vi "PicoScope2000aNearestSampleInterval.vi"(5 "Enabled array":i16[](array[numeric])=[0, 0, 0, 0, 0, 0, 0, 0, 0, 0], 6 "Acquisition Settings":T1 {"postTriggerSamples" format="%_6p"; "preTriggerSamples" format="%_6p"}, 8 "error in (no error)":errorcluster, 9 "roundFaster":bool, 10 "timeIntervalRequested":dbl format="%#6_6p", 11 "handle in":i16) -> (0 "error out":errorcluster, 1 "timebase":u32, 2 "timeIntervalAvailable":dbl format="%#6_6p", 3 "handle out":i16)   [LabVIEW 2010]
doc: "Calls Gettimebase function"
uses:
  ps2000a.dll
  shared/Acquisition Settings.ctl
panel:
  in  "Memory Segment":u32
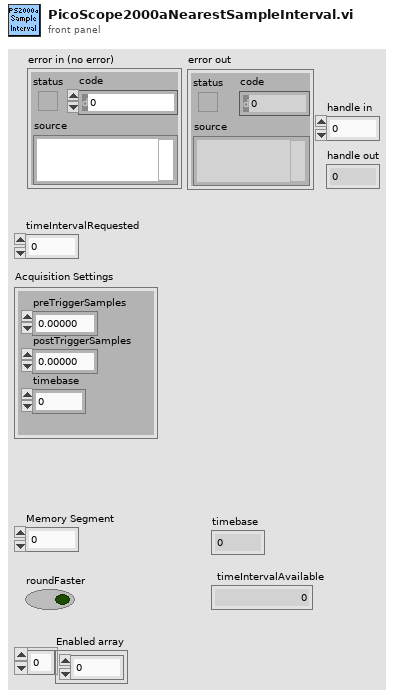
[diagram p1: front panel]
types:
  T1 = typedef "Acquisition Settings.ctl" = cluster{"preTriggerSamples":u64, "postTriggerSamples":u64, "timebase":u32}
  T2 = cluster{"status":bool, "code":u32, "source":string}
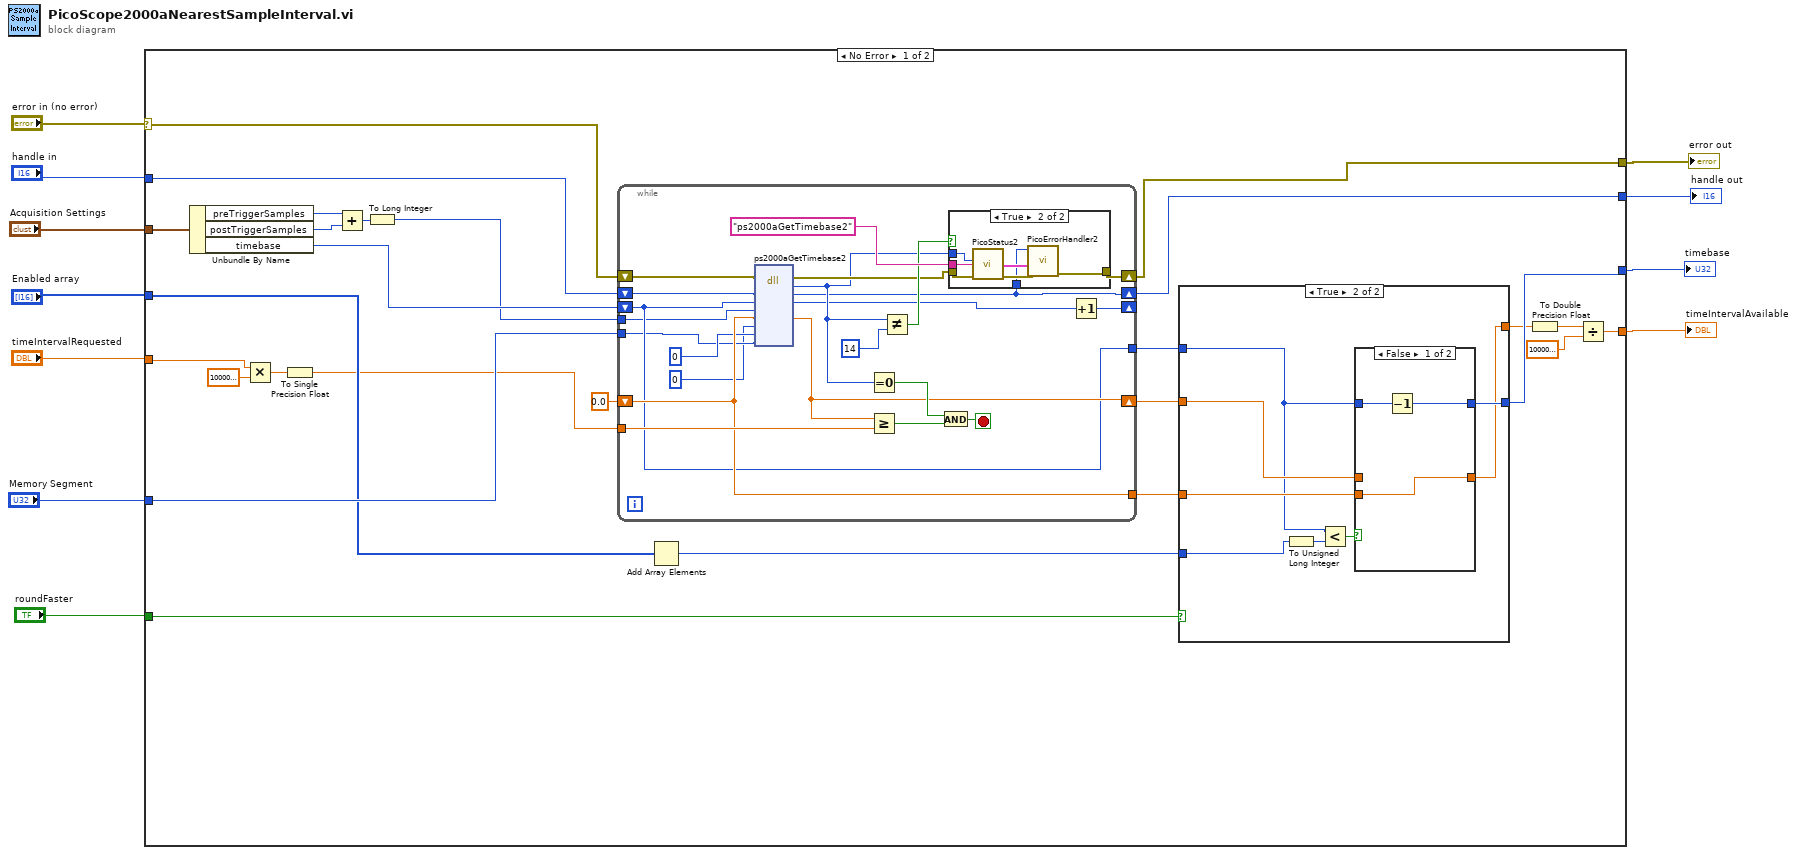
[diagram p0: block diagram]
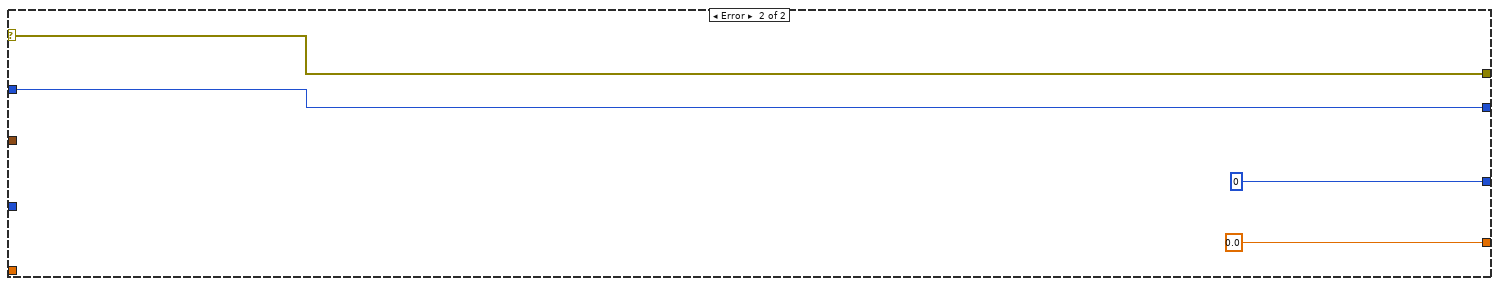
[diagram p5: hidden frame]
diagram:
  n1 = case shown="No Error" "error in (no error)" {
    selector: "error in (no error)" -> [w19 w87]
    tunnel: [w12 w87] -> w11
    tunnel: [w30 w86] -> w10
    tunnel: "handle in" -> [w31 w86]
    tunnel: "Enabled array" -> [w21 _]
    tunnel: "roundFaster" -> [w25 _]
    tunnel: "timeIntervalRequested" -> [w36 _]
    tunnel: [w22 u32 0 ("timebase")] -> w4
    tunnel: [w27 0.0 ("timeIntervalAvailable")] -> w3
    tunnel: "Acquisition Settings" -> [w32 _]
    tunnel: "Memory Segment" -> [w29 _]
    frame No Error {
      n2 = Unbundle By Name(w32) -> ("preTriggerSamples"=w34:u64, "postTriggerSamples"=w35:u64, "timebase"=w26:u32)
      n3 = Multiply(x=w36, y=1000000000.0) -> (x*y=w37:dbl)
      n4 = To Single Precision Float(number=w37) -> (single precision float=w18:sgl)
      n5 = Add(x=w34, y=w35) -> (x+y=w33:u64)
      n6 = To Long Integer(number=w33) -> (32bit integer=w20:i32)
      n7 = while {
        tunnel: w20 -> [w58]
        tunnel: w29 -> [w56]
        shift-right: [w54] -> w30
        shift-left: w31 -> [w61]
        shift-right: [w75] -> w12
        shift-left: w19 -> [w62]
        shift-right: [w73] -> _
        shift-left: w26 -> [w59]
        tunnel: w18 -> [w72]
        shift-right: [w64] -> w23
        shift-left: sgl 0.0 ("timeIntervalNanoseconds") -> [w60]
        tunnel: [w60] -> w24
        tunnel: [w59] -> w14
        stop <- w71 stop-if-true
        n8 = dll-call lib="ps2000a.dll" fn="ps2000aGetTimebase2"(error in=w62, "handle"=w61, "timebase"=w59, "noSamples"=w58, "timeIntervalNanoseconds"=w60, "oversample"=i16 0, "maxSamples"=0, "segmentIndex"=w56) -> (error out=w66:errorcluster, "PICO_STATUS"=w65:u32, "handle"=w54:i16, "timebase"=w63:u32, "timeIntervalNanoseconds"=w64:sgl)  [unwired: 6 in, 1 out]
        n9 = Equal To 0?(x=w65) -> (x = 0?=w69:bool)
        n10 = Greater Or Equal?(x=w64, y=w72) -> (x >= y?=w70:bool)
        n11 = Not Equal?(x=w65, y=u32 14) -> (x != y?=w67:bool)
        n12 = And(x=w69, y=w70) -> (x .and. y?=w71:bool)
        n13 = case shown="True" w67 {
          tunnel: w66 -> [w76 w83]
          tunnel: [w76 w79] -> w75
          tunnel: "ps2000aGetTimebase2" ("source") -> [_ w82]
          tunnel: w65 -> [_ w81]
          tunnel: w54 -> [_ w77]
          frame False {
          }
          frame True {
            n14 = call "PicoStatus2.vi"("PICO source"=w82, "Error in"=w83, "PICO STATUS"=w81) -> ("error out"=w80:errorcluster, "PICO_STATUS out"=w78:T2)  [unwired: 5 in]
            n15 = call "PicoErrorHandler2.vi"("error in (no error)"=w80, "PICO_STATUS in"=w78, "handle In"=w77) -> ("error out"=w79:errorcluster)  [unwired: 8 in]
          }
        }
        n16 = Increment(x=w63) -> (x+1=w73:u32)
      }
      n17 = Add Array Elements(numeric array=w21) -> (sum=w13:i16)
      n18 = case shown="True" w25 {
        tunnel: [w40 w47] -> w15
        tunnel: w24 -> [_ w46]
        tunnel: w23 -> [w40 w45]
        tunnel: [w39 w48] -> w22
        tunnel: w14 -> [w39 w43]
        tunnel: w13 -> [_ w41]
        frame False {
        }
        frame True {
          n19 = To Unsigned Long Integer(number=w41) -> (unsigned 32bit integer=w42:u32)
          n20 = Less?(x=w43, y=w42) -> (x < y?=w44:bool)
          n21 = case shown="False" w44 {
            tunnel: [w51 w53] -> w48
            tunnel: w43 -> [w50 w53]
            tunnel: [w49 w52] -> w47
            tunnel: w46 -> [w49 _]
            tunnel: w45 -> [_ w52]
            frame False {
              n22 = Decrement(x=w50) -> (x-1=w51:u32)
            }
            frame True {
            }
          }
        }
      }
      n23 = To Double Precision Float(number=w15) -> (double precision float=w16:dbl)
      n24 = Divide(x=w16, y=1000000000.0) -> (x/y=w27:dbl)
    }
    frame Error {
    }
  }
  "error out" <- w11
  "handle out" <- w10
  "timebase" <- w4
  "timeIntervalAvailable" <- w3
